vi "writeU8FIFO.vi"(8 "error in (no error)":errorcluster, 9 "Timeout":i32, 10 "Data":u8[](array[numeric]), 11 "MockDisplacementCommandFIFO in":refnum<class "MockDisplacementlCommandFIFO.lvclass">) -> (0 "error out":errorcluster, 2 "ElementsRemaining":u32, 3 "MockDisplacementCommandFIFO out":refnum<class "MockDisplacementlCommandFIFO.lvclass">)   [LabVIEW 2016, in "MockDisplacementlCommandFIFO.lvclass"]
uses:
  MockDisplacementlCommandFIFO.lvclass
  MockDisplacementlCommandFIFO.lvclass/MockDisplacementlCommandFIFO.ctl
  <vilib>/Utility/error.llb/Error Cluster From Error Code.vi
  <vilib>/rvi/errors/niLvFpgaAdjustHostInterfaceError.vi
  <vilib>/rvi/interface/nirviMethod/nirviMethod.xnode
  <vilib>/FPGAPlugInAG/Dynamic/niLvFpga_WriteFifo_Dynamic.vi
  <vilib>/rvi/errors/niLvFpgaMergeErrorWithErrorCode.vi
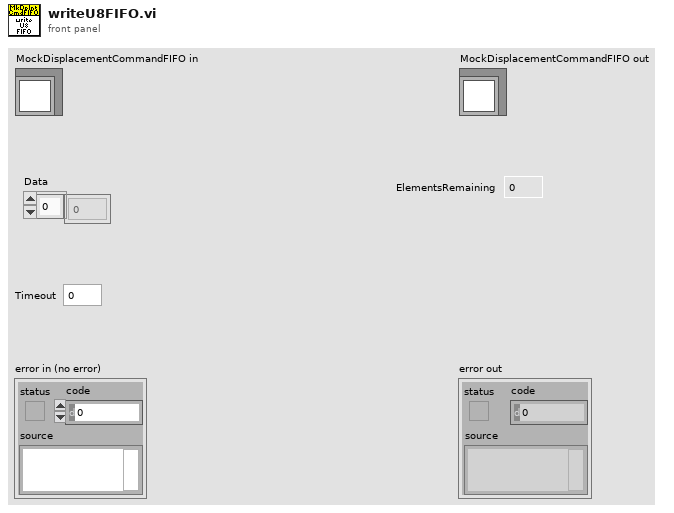
[diagram p1: front panel]
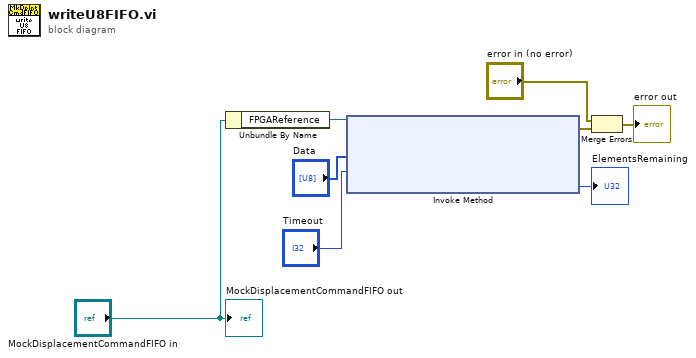
[diagram p0: block diagram]
diagram:
  n1 = Unbundle By Name("MockDisplacementCommandFIFO in") -> ("FPGAReference"=w7:refnum<k20>)
  n2 = xnode "Invoke Method"("FPGA VI Reference In"=w7, "Data"="Data", "Timeout (ms)"="Timeout") -> ("error out"=w3:errorcluster, "Empty Elements Remaining"=→"ElementsRemaining":u32)  [unwired: 1 in, 1 out]
  n3 = Merge Errors("error in (no error)", w3) -> (→"error out":errorcluster)
  "MockDisplacementCommandFIFO out" <- "MockDisplacementCommandFIFO in"
